vi "Auto Create String Type CaseStructure From ComboBox(冲突时的文件备份2013-05-03 10-26-16).vi"(8 "错误输入":errorcluster, 11 "组合框":string(combo)) -> (0 "错误输入（无错误）":errorcluster)   [LabVIEW 2012]
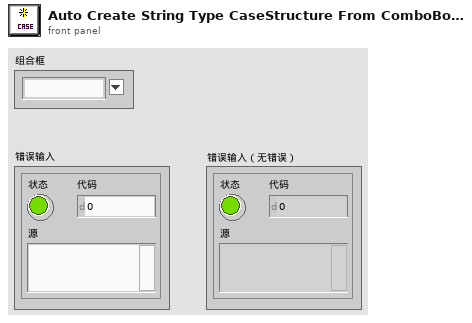
[diagram p1: front panel]
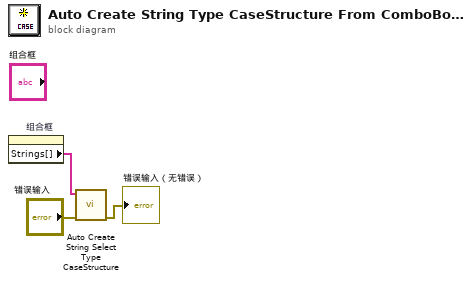
[diagram p0: block diagram]
diagram:
  n1 = property on="组合框" class="CmbBox"() -> ("Strings[]"=w3:string[])  [unwired: 2 in, 2 out]
  n2 = call "Auto Create String Select Type CaseStructure.vi"("错误输入（无错误）"="错误输入", "FrameNames"=w3) -> ("错误输出"=→"错误输入（无错误）":errorcluster)  [unwired: 9 in]
